vi "ventoinha cinematic.vi"() -> ()   [LabVIEW 2018]
panel:
  in  "stop":bool
  out "Time":dbl
  in  "GREEN Time":dbl
  in  "YELLOW Time":dbl
  in  "RED Time":dbl
  out "GREEN":bool
  out "YELLOW":bool
  out "RED":bool
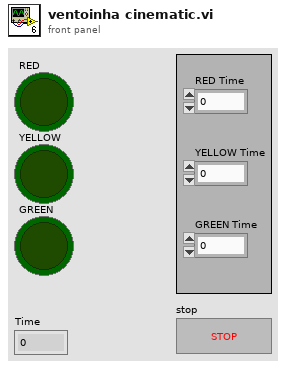
[diagram p1: front panel]
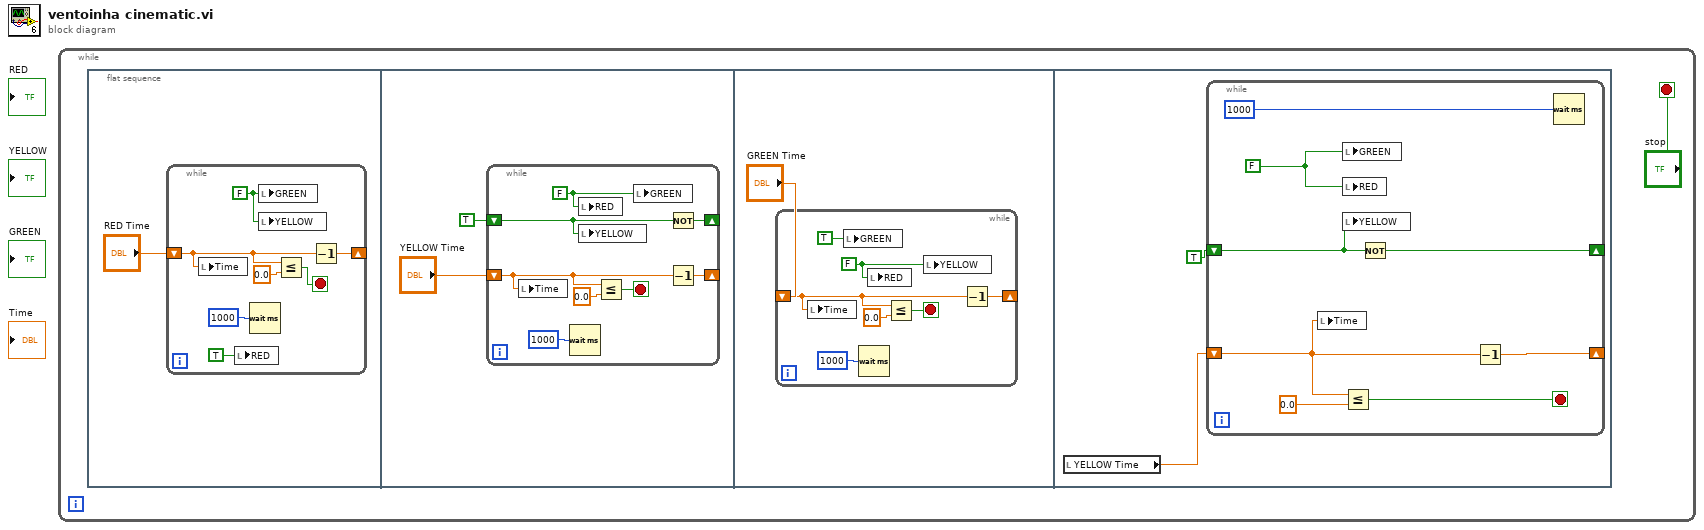
[diagram p0: block diagram]
diagram:
  n1 = while {
    stop <- "stop" stop-if-true
    n2 = flat-sequence {
      frame #0 {
        n3 = while {
          shift-right: [w7] -> _
          shift-left: "RED Time" -> [w5]
          stop <- w4 stop-if-true
          w9 = FALSE
          n4 = local write "Time"(w5) -> ()
          n5 = local write "RED"(TRUE) -> ()
          n6 = Wait (ms)(milliseconds to wait=u32 1000) -> ()  [unwired: 1 out]
          n7 = local write "GREEN"(w9) -> ()
          n8 = local write "YELLOW"(w9) -> ()
          n9 = Less Or Equal?(x=w5, y=0.0) -> (x <= y?=w4:bool)
          n10 = Decrement(x=w5) -> (x-1=w7:dbl)
        }
      }
      frame #1 {
        n11 = while {
          shift-right: [w19] -> _
          shift-left: "YELLOW Time" -> [w17]
          shift-right: [w13] -> _
          shift-left: TRUE -> [w12]
          stop <- w16 stop-if-true
          w14 = FALSE
          n12 = local write "Time"(w17) -> ()
          n13 = Wait (ms)(milliseconds to wait=u32 1000) -> ()  [unwired: 1 out]
          n14 = local write "RED"(w14) -> ()
          n15 = local write "YELLOW"(w12) -> ()
          n16 = Less Or Equal?(x=w17, y=0.0) -> (x <= y?=w16:bool)
          n17 = local write "GREEN"(w14) -> ()
          n18 = Not(x=w12) -> (.not. x?=w13:bool)
          n19 = Decrement(x=w17) -> (x-1=w19:dbl)
        }
      }
      frame #2 {
        n20 = while {
          shift-right: [w27] -> _
          shift-left: "GREEN Time" -> [w25]
          stop <- w24 stop-if-true
          w22 = FALSE
          n21 = local write "Time"(w25) -> ()
          n22 = local write "GREEN"(TRUE) -> ()
          n23 = Wait (ms)(milliseconds to wait=u32 1000) -> ()  [unwired: 1 out]
          n24 = local write "RED"(w22) -> ()
          n25 = Less Or Equal?(x=w25, y=0.0) -> (x <= y?=w24:bool)
          n26 = local write "YELLOW"(w22) -> ()
          n27 = Decrement(x=w25) -> (x-1=w27:dbl)
        }
      }
      frame #3 {
        n28 = local read "YELLOW Time"() -> (w28:dbl)
        n29 = while {
          shift-right: [w37] -> _
          shift-left: w28 -> [w35]
          shift-right: [w31] -> _
          shift-left: TRUE -> [w32]
          stop <- w30 stop-if-true
          w33 = FALSE
          n30 = local write "Time"(w35) -> ()
          n31 = local write "GREEN"(w33) -> ()
          n32 = local write "RED"(w33) -> ()
          n33 = local write "YELLOW"(w32) -> ()
          n34 = Less Or Equal?(x=w35, y=0.0) -> (x <= y?=w30:bool)
          n35 = Not(x=w32) -> (.not. x?=w31:bool)
          n36 = Decrement(x=w35) -> (x-1=w37:dbl)
          n37 = Wait (ms)(milliseconds to wait=u32 1000) -> ()  [unwired: 1 out]
        }
      }
    }
  }
